vi "CAN stop.vi"(4 "error in (no error)":errorcluster, 7 "CANopen in":refnum<class "CANopen.lvclass">) -> (0 "error out":errorcluster, 3 "CANopen out":refnum<class "CANopen.lvclass">)   [LabVIEW 2026, in "canopen_.lvlib" / "CANopen.lvclass"]
doc: "Stops the reading task and waits it is effectively stopped. Stopping is rarely needed because it is automatically done during \"CAN close\" but a pair of <B>CAN stop</B> and <B>CAN start</B> can be useful to reload the input map or the heartbeat table. The error cluster will return any error code caught by the task. If the CAN task has not been started before, the VI simply returns without error."
uses:
  CANopen.lvclass
  CANopen.lvclass/CANopen.ctl
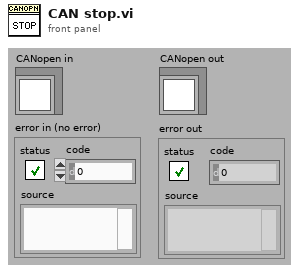
[diagram p1: front panel]
types:
  T1 = typedef "Semaphore RefNum" = refnum<k1>
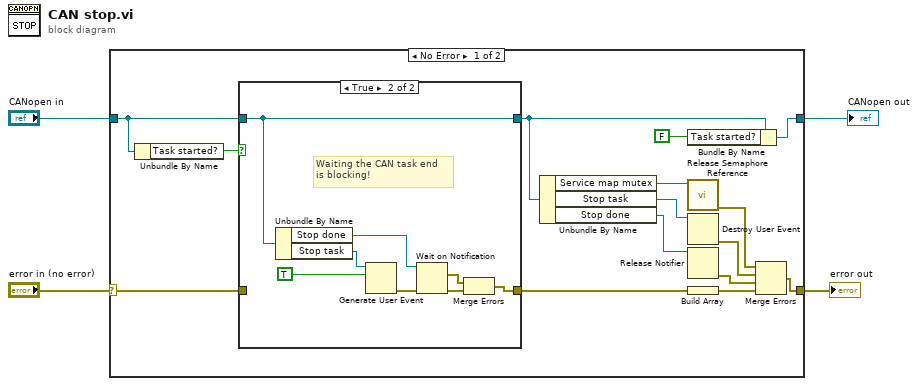
[diagram p0: block diagram]
diagram:
  n1 = case shown="No Error" "error in (no error)" {
    selector: "error in (no error)" -> [w17 w31]
    tunnel: "CANopen in" -> [w18 w30]
    tunnel: [w8 w31] -> w3
    tunnel: [w5 w30] -> w1
    frame No Error {
      n2 = Unbundle By Name(w18) -> ("Task started?"=w19:bool)
      n3 = case shown="True" w19 {
        tunnel: [w20 w27] -> w10
        tunnel: [w21 w24] -> w7
        tunnel: w18 -> [w21 w24]
        tunnel: w17 -> [w20 _]
        frame False {
        }
        frame True {
          # "Waiting the CAN task end\nis blocking!"
          n4 = Unbundle By Name(w24) -> ("Stop done"=w28:refnum<notifier>, "Stop task"=w29:refnum<user-event>)
          n5 = Generate User Event(user event=w29, event data cluster=TRUE ("event data")) -> (error out=w26:errorcluster)  [unwired: 2 in, 1 out]
          n6 = Wait on Notification(notifier=w28, error in (no error)=w26) -> (notification=w23:errorcluster, error out=w22:errorcluster)  [unwired: 4 out]
          n7 = Merge Errors(w23, w22) -> (w27:errorcluster)
        }
      }
      n8 = Unbundle By Name(w7) -> ("Service map mutex"=w14:T1, "Stop task"=w15:refnum<user-event>, "Stop done"=w16:refnum<notifier>)
      n9 = Bundle By Name(cluster=w7, "Task started?"=FALSE) -> (w5:refnum<class "CANopen.lvclass">)
      n10 = call <vilib>:"Release Semaphore Reference.vi"("semaphore"=w14) -> ("error out"=w13:errorcluster)  [unwired: 1 in, 9 out]
      n11 = Destroy User Event(user event=w15) -> (error out=w12:errorcluster)  [unwired: 1 in]
      n12 = Release Notifier(notifier=w16) -> (error out=w11:errorcluster)  [unwired: 1 in, 3 out]
      n13 = Build Array(w10) -> (w9:errorcluster[])
      n14 = Merge Errors(w13, w12, w11, w9) -> (w8:errorcluster)
    }
    frame Error {
    }
  }
  "error out" <- w3
  "CANopen out" <- w1
